vi "AvgFxp.vi"(11 "Analog Volt In [Int.]":i64) -> (3 "Analog Volt Out [FXP.]":fxp<+/-,22,5>)   [LabVIEW 2018, in "FPGA functions.lvlib"]
doc: "Covert from Integer value to scaled Fixed-point value between -10 to ~10 V.\n\nThe input is scaled sum of voltages from the moving sum filter."
uses:
  FPGA functions.lvlib
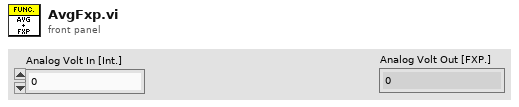
[diagram p1: front panel]
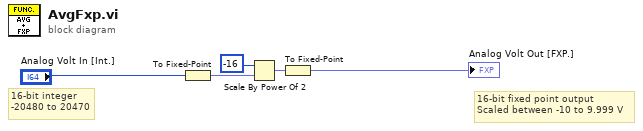
[diagram p0: block diagram]
diagram:
  # "16-bit fixed point output\nScaled between -10 to 9.999 V"
  # "16-bit integer \n-20480 to 20470"
  n1 = To Fixed-Point(number="Analog Volt In [Int.]") -> (fixed-point=w4:fxp<+/-,38,21>)  [unwired: 1 out]
  n2 = Scale By Power Of 2(n=-16, x=w4) -> (x*2^n=w3:fxp<+/-,38,21>)
  n3 = To Fixed-Point(number=w3) -> (fixed-point=→"Analog Volt Out [FXP.]":fxp<+/-,22,5>)  [unwired: 1 out]
